vi "MainForceSensors.vi"() -> ()   [LabVIEW 2017]
uses:
  <vilib>/Analysis/NI_AALBase.lvlib
  <vilib>/Analysis/baseanly.llb/A x Vector.vi
  <vilib>/DAQmx/read.llb/DAQmx Read (Analog 2D DBL NChan NSamp).vi
panel:
  out "TrialFileName":string
  out "condComb":string
  out "FbkDir":string
  out "FbkCond":string
  out "CtrlCond":string
  in  "ForceControl":bool
  in  "Horizontal VisualFBK":bool
  in  "udp_button switch":bool caption="BUTTON UDP switch"
  in  "invert FBK Direction":bool
  in  "Imposed Time":i32=2
  out "DataFilePAth":path
  out "recording state":bool
  in  "Data Saveing Dir":string="Z:\\Toma_S\\DataProofs\\Force\\"
  in  "Samples to Read":i32=50
  out "DataSaved":dbl[][][](array[numeric])
  out "timer":dbl
  out "Time":i32
  in  "n of trials":i32
  out "Block":i32
  out "trial":u8
  in  "UDP Sender Ip address":string="127.0.0.1"
  in  "Save data":bool caption="Off       On"
  out "SyncString":string
  out "SyncTime":string
  in  "bias transducers":bool
  out "F/T Values":dbl[][][](array[numeric])=[[[-0.0016047002615884648, 0.01962774474632563, 0.05388102532094477, -6.743846785846786e-05, 0.00032418926945717707, -0.0005535406771442331], [0.04658591023148378, 0.10359744995005873, 0.09177107845488962, 0.0007088752839781528, 0.0005091149263036229, -0.0001490476502194641], [0.038905158506793804, 0.041049406797413354, -0.2318981351133354, 0.0003706051814258798, 0.0003300945008706973, -0.0005507216127499452], [0.027342065946483203, 0.0063284743856839845, 0.011228207937424442, 0.0006610916509816831, 0.0007062586458297138, -0.00023219348927695451]], [[0.012798309188358076, 0.01092417773660311, 0.1272694001187903, -0.0001450092485733593, 0.0004738299906962181, -0.0007584704942989272], [0.012199878328640562, 0.0411633803945303, 0.03329774007675392, 0.0005124704259084759, 7.066848814634599e-05, 4.317642037141212e-05], [0.005299423293813158, -0.003370278256428499, -0.16521209929500077, 7.42094856124665e-05, 0.0005769248526913135, -0.0007510680850774225], [0.03254789740312213, 0.0032154344172637714, 0.06963187511481632, 0.00032399304516269787, -0.00019402019369577387, -0.0004224311720589758]], [[0.0017203445556565795, 0.023274075917015993, 0.039222554146342854, 5.02307106746716e-05, 5.724710676217142e-05, -0.0002546394943543632], [0.038336693856211336, 0.023469421725867298, 0.13860127402706493, 0.0014963025170351004, 0.0003243574753307975, -0.0003608981681178219], [0.027772762647286862, -0.038243515292141914, -0.13345045520840154, 9.913671599643043e-05, -0.0008372701697464751, -0.00023581040780558954], [-0.01973027621419694, -0.022088178591826317, 0.02227800713172409, 0.0001368646707220728, 0.00013841632865222076, 0.00021519155444430486]], [[0.005408013485119663, 0.025269142586546195, -0.011506447727556098, -2.86214169226201e-05, 0.00016210482159179708, -0.0003062657735645173], [-0.009895479653981737, 0.1206849398292366, 0.0745546395223249, 0.0010515350274939337, 0.0014625385879082678, -0.0001961015236909606], [0.016828393861908902, 0.009669503868452622, -0.050574579160010874, 7.920971038894653e-05, -0.0009941404806900968, -1.5702816965195018e-05], [-0.021115457140616637, -0.016045240815307994, -0.029438026591823107, 0.0008189640530756826, 0.0007296784451514024, -1.5204687815181738e-05]], [[0.01115190770446399, 0.03670379676857504, 0.053987135563857425, 8.217673960425931e-05, 0.00019271400758203553, -0.0004781661136652485], [0.03326798457303174, 0.010491146668883025, -0.05122056548368485, 0.0007232903324966133, -0.0008570729392138996, 7.55099522331733e-05], [-0.034266949639176605, -0.012241089683169651, -0.21451577126246754, 8.35103084577744e-05, 0.00021138857733046196, -0.0007826847508665894], [-0.006804253322395364, 0.006594023866956576, 0.03333855024951253, 0.0009013987634261645, 0.00042766532098932196, 0.00011011269207797162]], [[0.019268240656181098, 0.030977709668134738, 0.030124780747790923, 2.1615041776338006e-05, 0.00040297862709188077, -0.0002877869957582795], [0.1074302009600285, 0.06742696695484761, 0.06413956229885383, 0.0019178257669685405, -0.0004284434387014629, -0.00013452364101756628], [-0.027002371246654767, 0.009685154740743324, -0.05691670882486202, -0.00015283905251083568, 0.0007500746435299856, -0.00019091816134154659], [0.007730403501122321, 0.005287569848117169, 0.029276647486618575, 0.0007798916191205215, 0.00013216603713180397, -0.00034778124846752045]], [[0.011106503777328528, 0.022437646620986223, 0.06285462806248196, -4.220711725130722e-05, 0.0001071048785539649, -0.0003600837083180025], [-0.03585624769568089, 0.10159239430406058, 0.033044137367145114, 0.0011445878617654408, 0.001456551067444766, -4.409777862374308e-06], [-0.07814737243039128, 0.008376750644690014, 0.05992840508114507, -0.0006642828374729464, 0.000991671430226048, 0.00019742149066397614], [0.020635050521650898, -0.01908697049363589, -0.08002586349002709, 0.0007544280656719801, -8.343060734214193e-05, 2.672922988669045e-05]], [[0.004694513820669213, 0.019958593685490602, -0.05931338905984305, -0.00016146546080739402, 0.00031197690393288915, 0.00010907519352459618], [-0.034291165830070365, -0.027944921695361093, -0.008038070133952954, 9.719711647102313e-05, -0.0010158802770549697, 0.00035354049540800667], [-0.002764474884298997, 0.01715119342472284, 0.007148070321610785, 0.0003696295697706323, -0.0010631675337155033, -0.0011206366841255851], [-0.018376332726581426, -0.009490108392591609, -0.022941526529401835, -0.00016996172094216696, 0.00021113347550948776, -0.0002058381676953041]], [[0.02152190723156776, -0.012475360554489745, 0.014317154725799858, -0.00012821723872848102, -0.00010144804083618626, -0.0002670509161738814], [0.08287674571699581, 0.1102199258674346, 0.18993600502125194, 0.0013232448341828752, 0.0006198024650922631, -0.0004810808835829848], [-0.023481331116341198, 0.06279283487543294, -0.04140097663105311, 0.00010976198155341233, -0.0003293688251378183, -0.0009484470825381606], [0.0011932067018086917, -0.01345702513820748, 0.030125987341128455, -0.00011755926338180223, 0.0010380661254321998, -0.0002570805230206779]], [[0.013425963952264726, 0.030506283033742157, 0.1690182055294604, 0.0001222452324939653, 0.00040964377304742285, -0.0008257614692117129], [-0.029320557955479238, 0.12389666757935941, 0.059181057992992725, 0.0005116848191208073, 0.0008266184837498157, -8.966850322436495e-06], [0.04203919634544276, 0.05420012053008159, 0.023064952003368756, 0.0005140855843844264, -0.0010773765414121492, -0.001108730990409999], [-0.00821220027671831, -0.034998499190392836, -0.008470722665045245, -0.0004095754453320389, 0.0010658759922201459, 8.482416153973618e-05]]]
  in  "disconnect":bool
  out "subarray":dbl[][](array[numeric])=[[-0.0016047002615884648, 0.01962774474632563, 0.05388102532094477, -6.743846785846786e-05, 0.00032418926945717707, -0.0005535406771442331, 0.04658591023148378, 0.10359744995005873, 0.09177107845488962, 0.0007088752839781528, 0.0005091149263036229, -0.0001490476502194641, 0.038905158506793804, 0.041049406797413354, -0.2318981351133354, 0.0003706051814258798, 0.0003300945008706973, -0.0005507216127499452, 0.027342065946483203, 0.0063284743856839845, 0.011228207937424442, 0.0006610916509816831, 0.0007062586458297138, -0.00023219348927695451], [0.012798309188358076, 0.01092417773660311, 0.1272694001187903, -0.0001450092485733593, 0.0004738299906962181, -0.0007584704942989272, 0.012199878328640562, 0.0411633803945303, 0.03329774007675392, 0.0005124704259084759, 7.066848814634599e-05, 4.317642037141212e-05, 0.005299423293813158, -0.003370278256428499, -0.16521209929500077, 7.42094856124665e-05, 0.0005769248526913135, -0.0007510680850774225, 0.03254789740312213, 0.0032154344172637714, 0.06963187511481632, 0.00032399304516269787, -0.00019402019369577387, -0.0004224311720589758], [0.0017203445556565795, 0.023274075917015993, 0.039222554146342854, 5.02307106746716e-05, 5.724710676217142e-05, -0.0002546394943543632, 0.038336693856211336, 0.023469421725867298, 0.13860127402706493, 0.0014963025170351004, 0.0003243574753307975, -0.0003608981681178219, 0.027772762647286862, -0.038243515292141914, -0.13345045520840154, 9.913671599643043e-05, -0.0008372701697464751, -0.00023581040780558954, -0.01973027621419694, -0.022088178591826317, 0.02227800713172409, 0.0001368646707220728, 0.00013841632865222076, 0.00021519155444430486], [0.005408013485119663, 0.025269142586546195, -0.011506447727556098, -2.86214169226201e-05, 0.00016210482159179708, -0.0003062657735645173, -0.009895479653981737, 0.1206849398292366, 0.0745546395223249, 0.0010515350274939337, 0.0014625385879082678, -0.0001961015236909606, 0.016828393861908902, 0.009669503868452622, -0.050574579160010874, 7.920971038894653e-05, -0.0009941404806900968, -1.5702816965195018e-05, -0.021115457140616637, -0.016045240815307994, -0.029438026591823107, 0.0008189640530756826, 0.0007296784451514024, -1.5204687815181738e-05], [0.01115190770446399, 0.03670379676857504, 0.053987135563857425, 8.217673960425931e-05, 0.00019271400758203553, -0.0004781661136652485, 0.03326798457303174, 0.010491146668883025, -0.05122056548368485, 0.0007232903324966133, -0.0008570729392138996, 7.55099522331733e-05, -0.034266949639176605, -0.012241089683169651, -0.21451577126246754, 8.35103084577744e-05, 0.00021138857733046196, -0.0007826847508665894, -0.006804253322395364, 0.006594023866956576, 0.03333855024951253, 0.0009013987634261645, 0.00042766532098932196, 0.00011011269207797162], [0.019268240656181098, 0.030977709668134738, 0.030124780747790923, 2.1615041776338006e-05, 0.00040297862709188077, -0.0002877869957582795, 0.1074302009600285, 0.06742696695484761, 0.06413956229885383, 0.0019178257669685405, -0.0004284434387014629, -0.00013452364101756628, -0.027002371246654767, 0.009685154740743324, -0.05691670882486202, -0.00015283905251083568, 0.0007500746435299856, -0.00019091816134154659, 0.007730403501122321, 0.005287569848117169, 0.029276647486618575, 0.0007798916191205215, 0.00013216603713180397, -0.00034778124846752045], [0.011106503777328528, 0.022437646620986223, 0.06285462806248196, -4.220711725130722e-05, 0.0001071048785539649, -0.0003600837083180025, -0.03585624769568089, 0.10159239430406058, 0.033044137367145114, 0.0011445878617654408, 0.001456551067444766, -4.409777862374308e-06, -0.07814737243039128, 0.008376750644690014, 0.05992840508114507, -0.0006642828374729464, 0.000991671430226048, 0.00019742149066397614, 0.020635050521650898, -0.01908697049363589, -0.08002586349002709, 0.0007544280656719801, -8.343060734214193e-05, 2.672922988669045e-05], [0.004694513820669213, 0.019958593685490602, -0.05931338905984305, -0.00016146546080739402, 0.00031197690393288915, 0.00010907519352459618, -0.034291165830070365, -0.027944921695361093, -0.008038070133952954, 9.719711647102313e-05, -0.0010158802770549697, 0.00035354049540800667, -0.002764474884298997, 0.01715119342472284, 0.007148070321610785, 0.0003696295697706323, -0.0010631675337155033, -0.0011206366841255851, -0.018376332726581426, -0.009490108392591609, -0.022941526529401835, -0.00016996172094216696, 0.00021113347550948776, -0.0002058381676953041], [0.02152190723156776, -0.012475360554489745, 0.014317154725799858, -0.00012821723872848102, -0.00010144804083618626, -0.0002670509161738814, 0.08287674571699581, 0.1102199258674346, 0.18993600502125194, 0.0013232448341828752, 0.0006198024650922631, -0.0004810808835829848, -0.023481331116341198, 0.06279283487543294, -0.04140097663105311, 0.00010976198155341233, -0.0003293688251378183, -0.0009484470825381606, 0.0011932067018086917, -0.01345702513820748, 0.030125987341128455, -0.00011755926338180223, 0.0010380661254321998, -0.0002570805230206779], [0.013425963952264726, 0.030506283033742157, 0.1690182055294604, 0.0001222452324939653, 0.00040964377304742285, -0.0008257614692117129, -0.029320557955479238, 0.12389666757935941, 0.059181057992992725, 0.0005116848191208073, 0.0008266184837498157, -8.966850322436495e-06, 0.04203919634544276, 0.05420012053008159, 0.023064952003368756, 0.0005140855843844264, -0.0010773765414121492, -0.001108730990409999, -0.00821220027671831, -0.034998499190392836, -0.008470722665045245, -0.0004095754453320389, 0.0010658759922201459, 8.482416153973618e-05]]
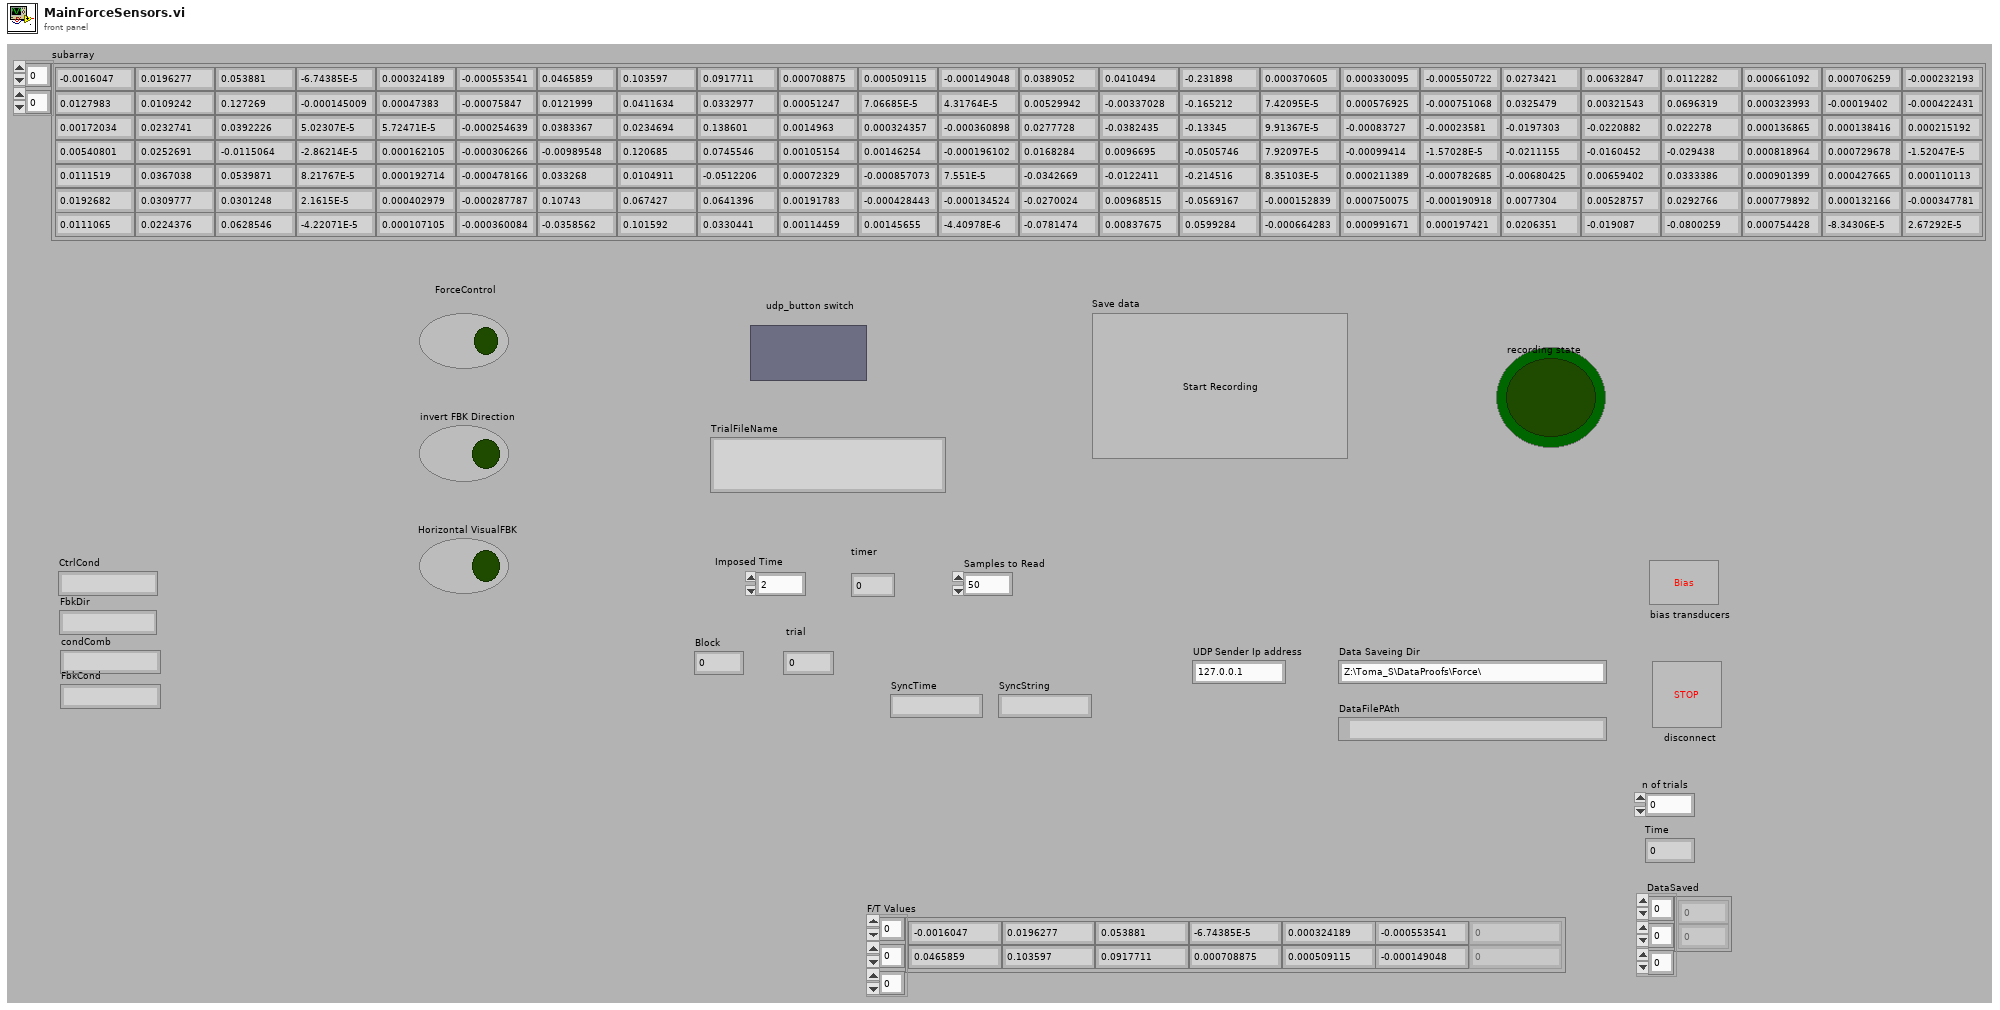
[diagram p1: front panel]
types:
  T1 = enum16{"open", "replace", "create", "open or create", "replace or create", "replace or create with confirmation"}
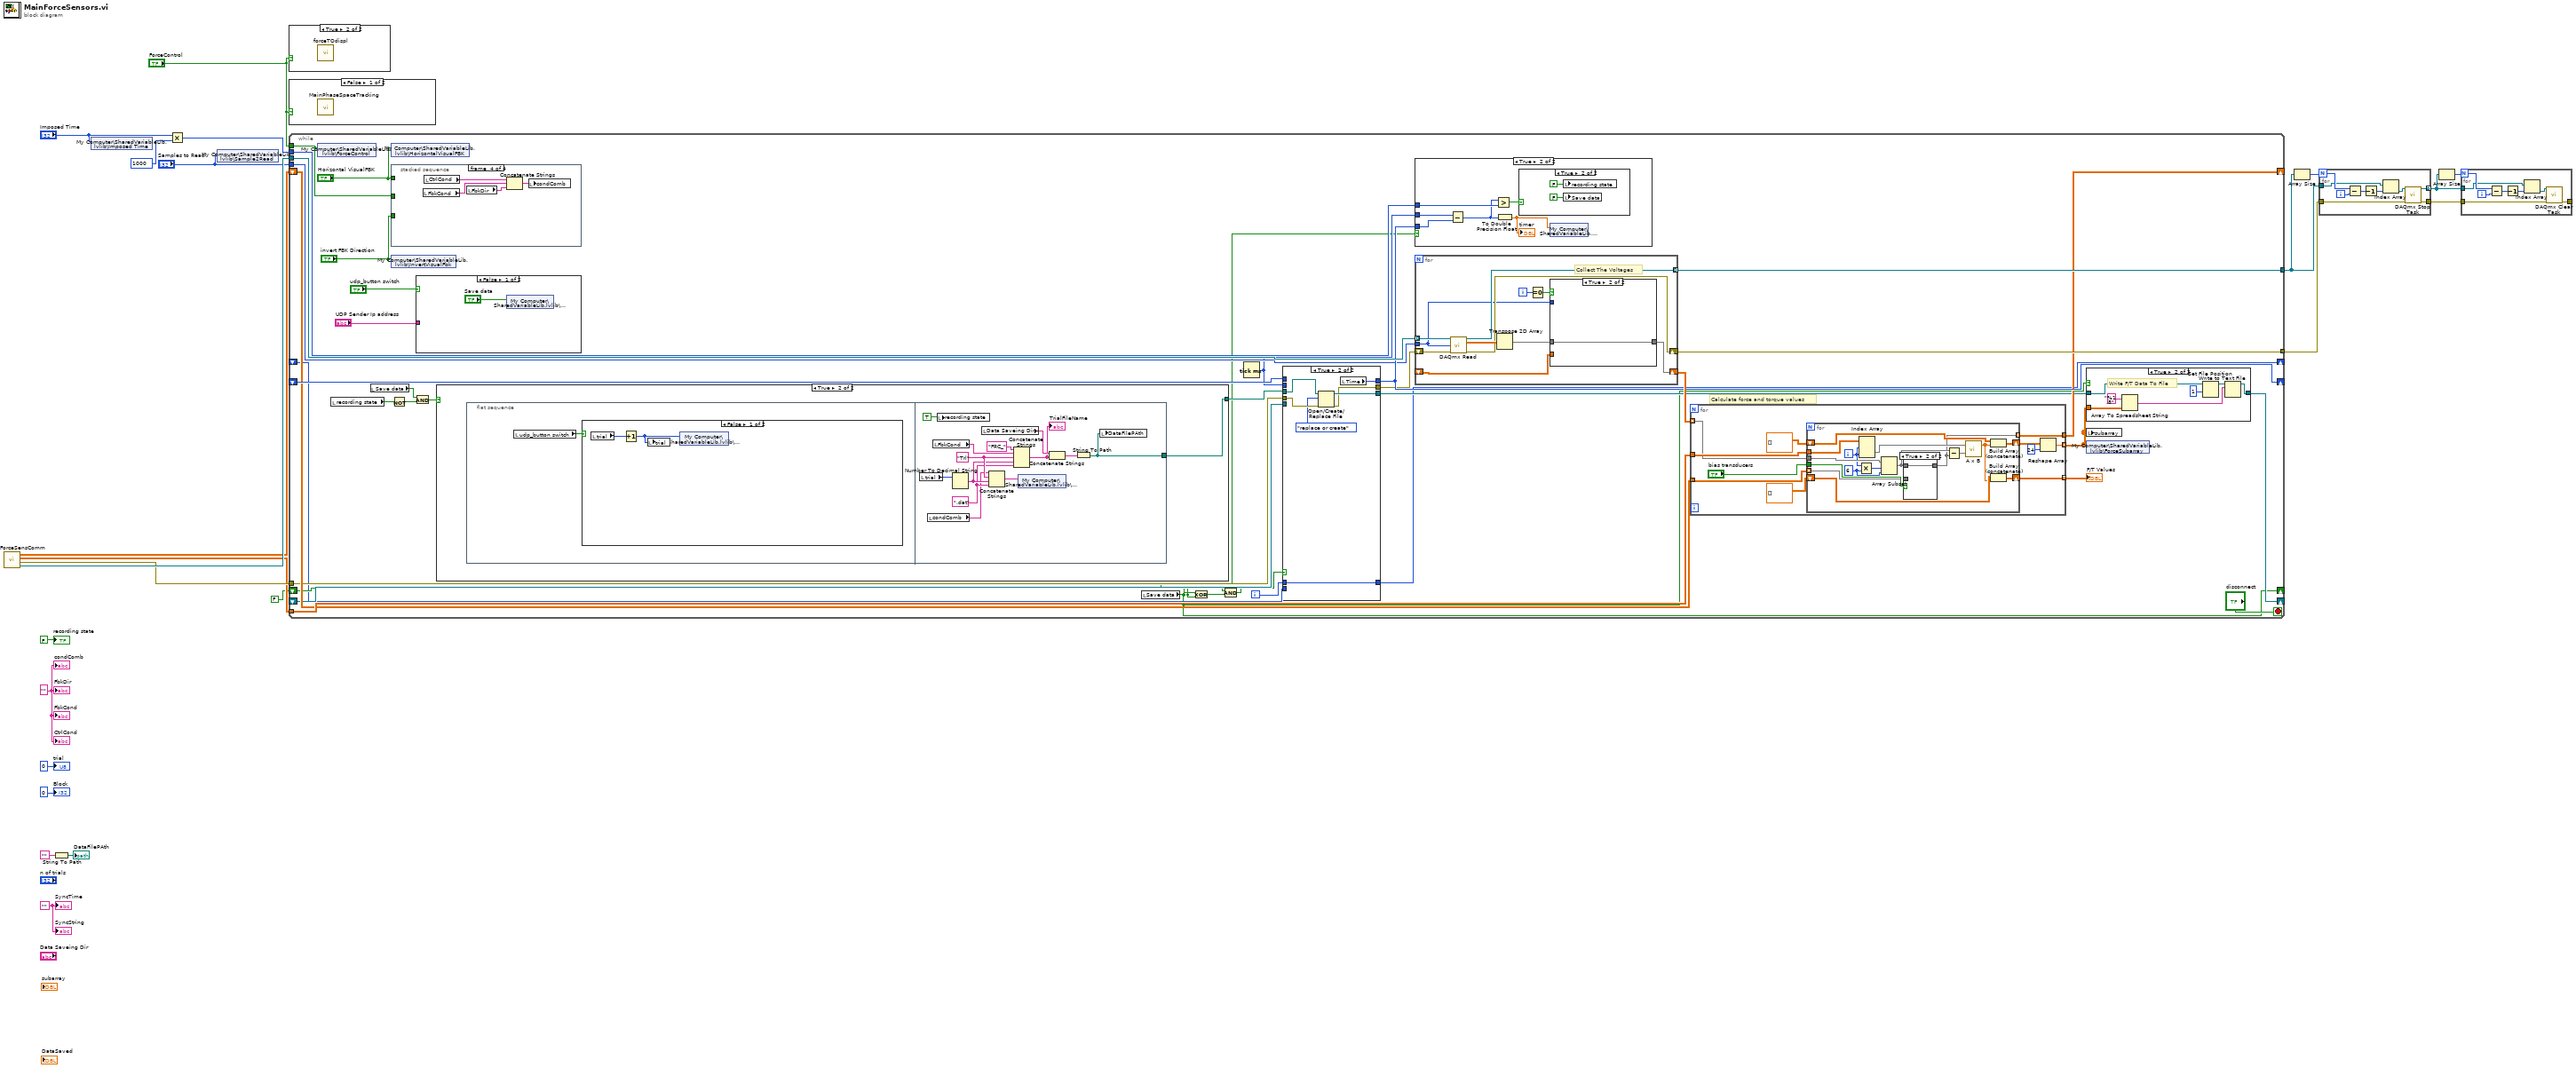
[diagram p0: block diagram]
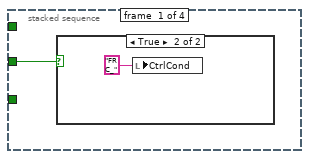
[diagram p4: hidden frame]
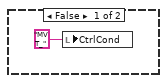
[diagram p5: hidden frame]
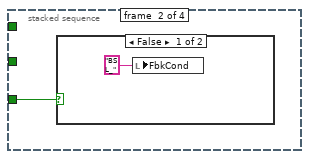
[diagram p6: hidden frame]
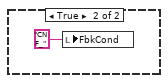
[diagram p7: hidden frame]
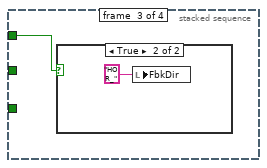
[diagram p8: hidden frame]
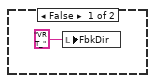
[diagram p9: hidden frame]
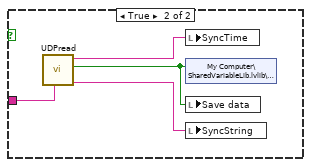
[diagram p10: hidden frame]
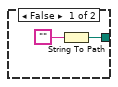
[diagram p11: hidden frame]
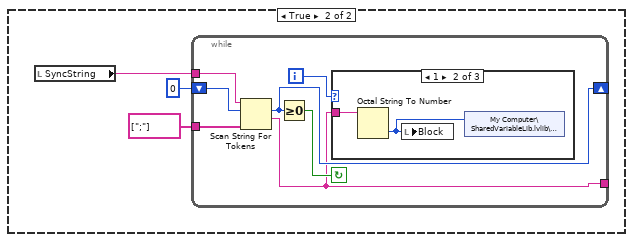
[diagram p12: hidden frame]
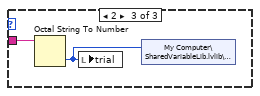
[diagram p14: hidden frame]
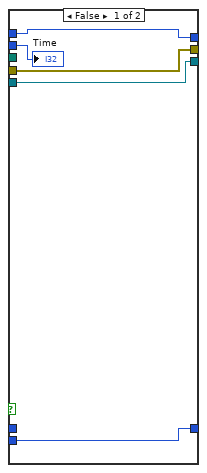
[diagram p18: hidden frame]
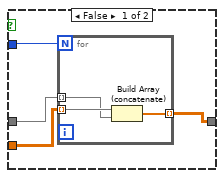
[diagram p20: hidden frame]
diagram:
  w1 = ""
  w17 = ""
  n1 = call "ForceSensComm.vi"() -> ("Daq Array"=w15:refnum<k21>[], "error out"=w14:errorcluster, "Array1"=w12:sgl[][][], "Array"=w13:dbl[][])  [unwired: 8 out]
  n2 = String To Path(string="") -> (path=→"DataFilePAth":path)
  n3 = shared-variable "My Computer\\SharedVariableLib.lvlib\\Imposed Time"("Imposed Time") -> ()  [unwired: 1 in, 1 out]
  n4 = Multiply(x="Imposed Time", y=u16 1000) -> (x*y=w9:i32)
  n5 = shared-variable "My Computer\\SharedVariableLib.lvlib\\Sample2Read"("Samples to Read") -> ()  [unwired: 1 in, 1 out]
  n6 = case shown="True" "ForceControl" {
    frame False {
    }
    frame True {
      n7 = call "forceTOdispl.vi"() -> ()  [unwired: 11 in]
    }
  }
  n8 = case shown="False" "ForceControl" {
    frame False {
      n9 = call "MainPhaseSpaceTracking.vi"() -> ()  [unwired: 1 in]
    }
    frame True {
    }
  }
  n10 = while {
    tunnel: w15 -> [w58]
    tunnel: w12 -> [w59]
    tunnel: w14 -> [w48]
    tunnel: [w56] -> w19
    tunnel: "Samples to Read" -> [w51]
    shift-right: [w53] -> _
    shift-left: _ -> [w57]
    tunnel: [w55] -> w20
    shift-right: [w29] -> _
    shift-left: _ -> [w32]
    shift-right: [w46] -> _
    shift-left: w13 -> [w54]
    tunnel: w9 -> [w50]
    shift-right: [w45] -> _
    shift-left: _ -> [w43]
    shift-right: [w30] -> _
    shift-left: FALSE -> [w41]
    tunnel: "ForceControl" -> [w25]
    i -> [w49]
    stop <- "disconnect" stop-if-true
    # "Calculate force and torque values"
    n11 = shared-variable "My Computer\\SharedVariableLib.lvlib\\ForceControl"(w25) -> ()  [unwired: 1 in, 1 out]
    n12 = local read "recording state"() -> (w38:bool)
    n13 = local read "Save data"() -> (w36:bool)
    n14 = shared-variable "My Computer\\SharedVariableLib.lvlib\\HorizontalVisualFBK"("Horizontal VisualFBK") -> ()  [unwired: 1 in, 1 out]
    n15 = stacked-sequence {
      tunnel: w25 -> [w61 _ _ _]
      tunnel: "invert FBK Direction" -> [_ w64 _ _]
      tunnel: "Horizontal VisualFBK" -> [_ _ w67 _]
      frame #0 {
        n16 = case shown="True" w61 {
          frame False {
            n17 = local write "CtrlCond"("MVT_") -> ()
          }
          frame True {
            n18 = local write "CtrlCond"("FRC_") -> ()
          }
        }
      }
      frame #1 {
        n19 = case shown="False" w64 {
          frame False {
            n20 = local write "FbkCond"("BSL_") -> ()
          }
          frame True {
            n21 = local write "FbkCond"("CNF_") -> ()
          }
        }
      }
      frame #2 {
        n22 = case shown="True" w67 {
          frame False {
            n23 = local write "FbkDir"("VRT_") -> ()
          }
          frame True {
            n24 = local write "FbkDir"("HOR_") -> ()
          }
        }
      }
      frame #3 {
        n25 = local read "FbkCond"() -> (w72:string)
        n26 = local read "CtrlCond"() -> (w73:string)
        n27 = local read "FbkDir"() -> (w71:string)
        n28 = Concatenate Strings(w73, w72, w71) -> (w70:string)
        n29 = local write "condComb"(w70) -> ()
      }
    }
    n30 = shared-variable "My Computer\\SharedVariableLib.lvlib\\InvertVisualFbk"("invert FBK Direction") -> ()  [unwired: 1 in, 1 out]
    n31 = Not(x=w38) -> (.not. x?=w37:bool)
    n32 = And(x=w36, y=w37) -> (x .and. y?=w26:bool)
    n33 = case shown="False" "udp_button switch" {
      tunnel: "UDP Sender Ip address" -> [_ w78]
      frame False {
        n34 = shared-variable "My Computer\\SharedVariableLib.lvlib\\StartRec"("Save data") -> ()  [unwired: 1 in, 1 out]
      }
      frame True {
        n35 = call "UDPread.vi"("Sender Ip address"=w78) -> ("UDP read string"=w77:string, "recording Switch"=w75:bool, "udp time of received"=w76:string)  [unwired: 8 in]
        n36 = local write "SyncTime"(w76) -> ()
        n37 = shared-variable "My Computer\\SharedVariableLib.lvlib\\StartRec"(w75) -> ()  [unwired: 1 in, 1 out]
        n38 = local write "Save data"(w75) -> ()
        n39 = local write "SyncString"(w77) -> ()
      }
    }
    n40 = case shown="True" w26 {
      tunnel: [w79 w81] -> w34
      frame False {
        n41 = String To Path(string="") -> (path=w79:path)
      }
      frame True {
        n42 = flat-sequence {
          tunnel: [w109] -> w81
          frame #0 {
            n43 = local read "udp_button switch"() -> (w82:bool)
            n44 = case shown="False" w82 {
              frame False {
                n45 = local read "trial"() -> (w84:u8)
                n46 = Increment(x=w84) -> (x+1=w83:u8)
                n47 = local write "trial"(w83) -> ()
                n48 = shared-variable "My Computer\\SharedVariableLib.lvlib\\Trial num"(w83) -> ()  [unwired: 1 in, 1 out]
              }
              frame True {
                n49 = local read "SyncString"() -> (w85:string)
                n50 = while {
                  tunnel: string[] [";"] ("Array") -> [w94]
                  tunnel: w85 -> [w93]
                  shift-right: [w89] -> _
                  shift-left: 0 -> [w92]
                  tunnel: [w88] -> _
                  i -> [w90]
                  stop <- w91 continue-if-true
                  n51 = Scan String For Tokens(6:w94, 8:w92, 9:w93) -> (1:w88:string, 2:w89:i32)  [unwired: 5 out]
                  n52 = Greater Or Equal To 0?(x=w89) -> (x >= 0?=w91:bool)
                  n53 = case shown="1" w90 {
                    tunnel: w88 -> [_ w96 w98]
                    frame 0, Default {
                    }
                    frame 1 {
                      n54 = Octal String To Number(4:w96) -> (0:w95:u32)  [unwired: 3 out]
                      n55 = local write "Block"(w95) -> ()
                      n56 = shared-variable "My Computer\\SharedVariableLib.lvlib\\Block num"(w95) -> ()  [unwired: 1 in, 1 out]
                    }
                    frame 2 {
                      n57 = Octal String To Number(4:w98) -> (0:w97:u32)  [unwired: 3 out]
                      n58 = local write "trial"(w97) -> ()
                      n59 = shared-variable "My Computer\\SharedVariableLib.lvlib\\Trial num"(w97) -> ()  [unwired: 1 in, 1 out]
                    }
                  }
                }
              }
            }
          }
          frame #1 {
            w105 = "Trl"
            w103 = ".dat"
            n60 = local read "trial"() -> (w111:u8)
            n61 = local read "condComb"() -> (w101:string)
            n62 = local read "FbkCond"() -> (w99:string)
            n63 = local write "recording state"(TRUE) -> ()
            n64 = Number To Decimal String(number=w111) -> (decimal integer string=w104:string)  [unwired: 1 out]
            n65 = local read "Data Saveing Dir"() -> (w108:string)
            n66 = Concatenate Strings(w101, w105, w104, w103) -> (w102:string)
            n67 = Concatenate Strings("FRC_" ("condComb"), w99, w105, w104, w103) -> (w106:string)
            "TrialFileName" <- w106
            n68 = shared-variable "My Computer\\SharedVariableLib.lvlib\\FileName"(w102) -> ()  [unwired: 1 in, 1 out]
            n69 = Concatenate Strings(w108, w106) -> (w107:string)
            n70 = String To Path(string=w107) -> (path=w109:path)
            n71 = local write "DataFilePAth"(w109) -> ()
          }
        }
      }
    }
    n72 = local read "Save data"() -> (w30:bool)
    n73 = Exclusive Or(1:w30, 2:w41) -> (0:w42:bool)
    n74 = Compound Arithmetic op=AND(w30, w42) -> (w35:bool)
    n75 = Tick Count (ms)() -> (millisecond timer value=w39:u32)
    n76 = case shown="True" w35 {
      tunnel: [w132 w135] -> w53
      tunnel: w57 -> [w132 _]
      tunnel: w49 -> [_ w139]
      tunnel: [w131 w139] -> w29
      tunnel: w32 -> [w131 _]
      tunnel: [w130 w138] -> w44
      tunnel: w43 -> [w130 _]
      tunnel: w48 -> [w129 w137]
      tunnel: [w129 w136] -> w47
      tunnel: w39 -> [w128 _]
      tunnel: w34 -> [_ w134]
      frame False {
        "Time" <- w128
      }
      frame True {
        n77 = Open/Create/Replace File(file path (use dialog)=w134, error in=w137, operation (0:open)=T1."replace or create") -> (refnum out=w138:refnum<file>, error out=w136:errorcluster)  [unwired: 4 out]
        n78 = local read "Time"() -> (w135:i32)
      }
    }
    n79 = case shown="True" w30 {
      tunnel: w39 -> [_ w123]
      tunnel: w53 -> [_ w124]
      tunnel: w50 -> [_ w125]
      frame False {
      }
      frame True {
        n80 = Subtract(x=w123, y=w124) -> (x-y=w122:u32)
        n81 = Greater?(x=w122, y=w125) -> (0:w121:bool)
        n82 = To Double Precision Float(number=w122) -> (double precision float=w120:dbl)
        "timer" <- w120
        n83 = case shown="True" w121 {
          frame False {
          }
          frame True {
            n84 = local write "recording state"(FALSE) -> ()
            n85 = local write "Save data"(FALSE ("Save data")) -> ()
          }
        }
        n86 = shared-variable "My Computer\\SharedVariableLib.lvlib\\Timer"(w120) -> ()  [unwired: 1 in, 1 out]
      }
    }
    n87 = for {
      tunnel: w58 -> [w179] mode=indexing
      shift-right: [w176] -> w56
      shift-left: w47 -> [w178]
      shift-right: [w173] -> w60
      shift-left: _ -> [w171]
      tunnel: w51 -> [w169]
      tunnel: [w170] -> w55 mode=indexing
      i -> [w175]
      # "Collect The Voltages"
      n88 = call-poly <vilib>:"DAQmx Read.vi"("task/channels in"=w179, "number of samples per channel"=w169, "error in"=w178) -> ("task out"=w170:refnum<k21>, "data"=w177:dbl[][], "error out"=w176:errorcluster)  [unwired: 10 out]
      n89 = Transpose 2D Array(2D array=w177) -> (transposed array=w172:dbl[][])
      n90 = Equal To 0?(x=w175) -> (x = 0?=w174:bool)
      n91 = case shown="True" w174 {
        tunnel: [w181 w187] -> w173
        tunnel: w172 -> [w182 w187]
        tunnel: w171 -> [w183 _]
        tunnel: w169 -> [w180 _]
        frame False {
          n92 = for {
            N: w180 -> [_]
            tunnel: w183 -> [w186] mode=indexing
            tunnel: w182 -> [w185] mode=indexing
            tunnel: [w184] -> w181 mode=indexing
            n93 = Build Array (concatenate)(w186, w185) -> (w184:dbl[])
          }
        }
        frame True {
        }
      }
    }
    n94 = for {
      tunnel: w60 -> [w149] mode=indexing
      tunnel: w59 -> [w150]
      tunnel: [w146] -> w40 mode=indexing
      tunnel: [w141] -> w28 mode=indexing
      tunnel: w54 -> [w142]
      tunnel: [w143] -> w46
      n95 = for {
        tunnel: w150 -> [w162]
        tunnel: w149 -> [w163]
        tunnel: w142 -> [w153] mode=indexing
        shift-right: [w158] -> w140
        shift-left: dbl[][] [] -> [w160]
        shift-right: [w159] -> w146
        shift-left: sgl[][] [] -> [w161]
        tunnel: "bias transducers" -> [w154]
        tunnel: [w151] -> w143 mode=indexing
        i -> [w157]
        w165 = 6
        n96 = Multiply(x=w157, y=w165) -> (x*y=w166:i32)
        n97 = Index Array(array=w162, index (dim 0)=w157) -> (element=w164:sgl[][])  [unwired: 2 in]
        n98 = Array Subset(array=w163, index=w166, length=w165) -> (w152:dbl[])
        n99 = case shown="True" w154 {
          tunnel: w153 -> [w167 _]
          tunnel: [w167 w168] -> w151
          tunnel: w152 -> [_ w168]
          frame False {
          }
          frame True {
          }
        }
        n100 = Subtract(x=w152, y=w151) -> (x-y=w156:dbl[])
        n101 = call-poly <vilib>:"A x B.vi"("Vector"=w156, "A"=w164) -> ("A x Vector"=w155:dbl[])  [unwired: 1 out]
        n102 = Build Array (concatenate)(w160, w155) -> (w158:dbl[][])
        n103 = Build Array (concatenate)(w161, w155) -> (w159:dbl[][])
      }
      n104 = Reshape Array(w140, 24 ("dimension size")) -> (w141:dbl[])
    }
    "F/T Values" <- w40
    n105 = case shown="True" w30 {
      tunnel: w28 -> [_ w113]
      tunnel: [w112 w119] -> w45
      tunnel: w44 -> [w112 w118]
      frame False {
      }
      frame True {
        # "Write F/T Data To File"
        n106 = Array To Spreadsheet String(array=w113, 3:"%1.8" ("format string")) -> (spreadsheet string=w115:string)  [unwired: 1 out]
        n107 = Set File Position(refnum=w118, from (0:start)=1) -> (refnum out=w116:refnum<file>)  [unwired: 1 in, 2 out]
        n108 = Write to Text File(file (use dialog)=w116, text=w115) -> (refnum out=w119:refnum<file>)  [unwired: 1 in, 3 out]
      }
    }
    n109 = local write "subarray"(w28) -> ()
    n110 = shared-variable "My Computer\\SharedVariableLib.lvlib\\ForceSubarray"(w28) -> ()  [unwired: 1 in, 1 out]
  }
  n111 = Array Size(array=w20) -> (size(s)=w18:i32)
  n112 = for {
    N: w18 -> [w196]
    tunnel: w20 -> [w191]
    tunnel: w19 -> [w192]
    tunnel: [w189] -> w22
    tunnel: [w188] -> w21 mode=indexing
    i -> [w195]
    n113 = Subtract(x=w196, y=w195) -> (x-y=w194:i32)
    n114 = Decrement(x=w194) -> (x-1=w190:i32)
    n115 = Index Array(array=w191, index=w190) -> (element=w193:refnum<k21>)
    n116 = call <vilib>:"DAQmx Stop Task.vi"("task/channels in"=w193, "error in"=w192) -> ("task out"=w188:refnum<k21>, "error out"=w189:errorcluster)  [unwired: 12 out]
  }
  n117 = Array Size(array=w21) -> (size(s)=w23:i32)
  n118 = for {
    N: w23 -> [w204]
    tunnel: w21 -> [w199]
    tunnel: w22 -> [w200]
    tunnel: [w197] -> _
    i -> [w203]
    n119 = Subtract(x=w204, y=w203) -> (x-y=w202:i32)
    n120 = Decrement(x=w202) -> (x-1=w198:i32)
    n121 = Index Array(array=w199, index=w198) -> (element=w201:refnum<k21>)
    n122 = call <vilib>:"DAQmx Clear Task.vi"("task in"=w201, "error in"=w200) -> ("error out"=w197:errorcluster)  [unwired: 13 out]
  }
  "SyncTime" <- w17
  "SyncString" <- w17
  "trial" <- 0
  "Block" <- 0
  "recording state" <- FALSE
  "CtrlCond" <- w1
  "FbkCond" <- w1
  "FbkDir" <- w1
  "condComb" <- w1
